vi "Get-control.vi"(8 "error in (no error)":errorcluster, 10 "Control name":T1, 11 "Panes in":T2) -> (0 "error out":errorcluster, 2 "Ctl Refnum":refnum<vi>, 3 "Panes out":T2)   [LabVIEW 2013, in "HardwareCharacterization.lvlib" / "HC-UI.lvclass"]
uses:
  HC-UI.lvclass
  Panes-reference.ctl
  Control-names.ctl
  HC-UI.lvclass/HC-UI.ctl
  Read Controls lib.vi
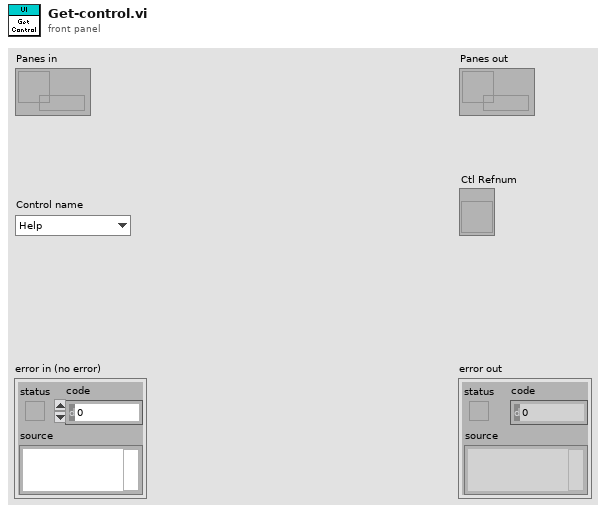
[diagram p1: front panel]
types:
  T1 = typedef "HardwareCharacterization.lvlib/HC-UI.lvclass/Control-names.ctl" = enum16{"Help", "Status", "Load configuration", "Save configuration", "Activate", "Start", "Stop", "Options"}
  T2 = typedef "HardwareCharacterization.lvlib/HC-UI.lvclass/Panes-reference.ctl" = refnum<data-value>
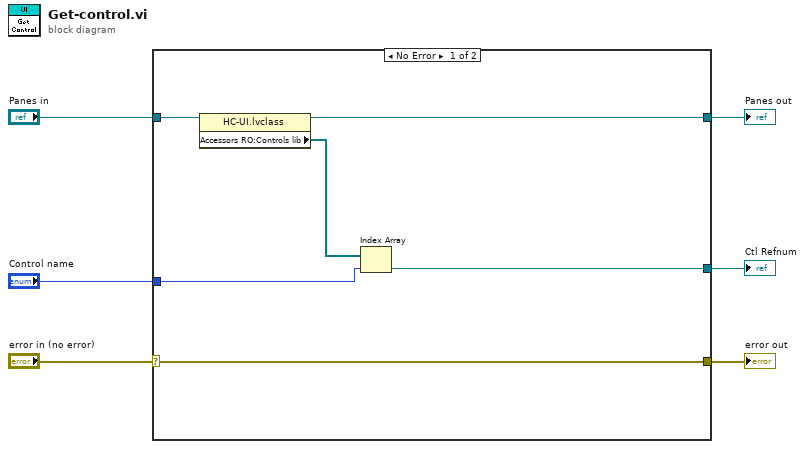
[diagram p0: block diagram]
diagram:
  n1 = case shown="No Error" "error in (no error)" {
    selector: "error in (no error)" -> [w7 w13]
    tunnel: [w7 w13] -> w5
    tunnel: [w11 w14] -> w3
    tunnel: "Panes in" -> [w12 w14]
    tunnel: "Control name" -> [w9 _]
    tunnel: [w8 _] -> w1
    frame No Error {
      n2 = property class="HC-UI.lvclass"(reference=w12) -> (reference out=w11:T2, "Accessors RO:Controls lib"=w10:refnum<vi>[])  [unwired: 1 in, 1 out]
      n3 = Index Array(array=w10, index=w9) -> (element=w8:refnum<vi>)
    }
    frame Error {
    }
  }
  "error out" <- w5
  "Panes out" <- w3
  "Ctl Refnum" <- w1
